vi "saveSettings.vi"(8 "error in (no error)":errorcluster, 11 "TaskRef in":refnum<vi>) -> (0 "error out":errorcluster, 3 "TaskRef out":refnum<vi>)   [LabVIEW 2015, in "pdbm_tasks.lvlib"]
doc: "saves current value of controls on VI to file. The setting file is placed in Config folder in application root folder and named as below rule thumb: <b><VI_Name>_setting.xml</b>"
uses:
  pdbm_tasks.lvlib
  <vilib>/Utility/error.llb/DialogType.ctl
  <vilib>/NI/GXML/Utility VIs/Concatenate GXML Strings.vi
  <vilib>/NI/GXML/Generator.vi
  <vilib>/NI/GXML/Write XML to File.vi
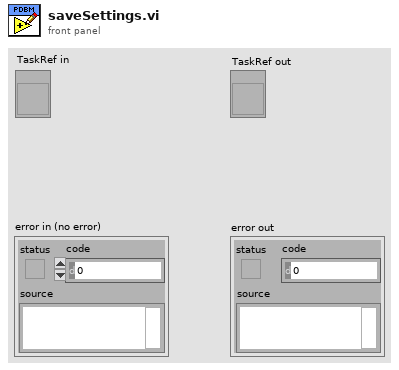
[diagram p1: front panel]
types:
  T1 = typedef "DialogType.ctl" = u16
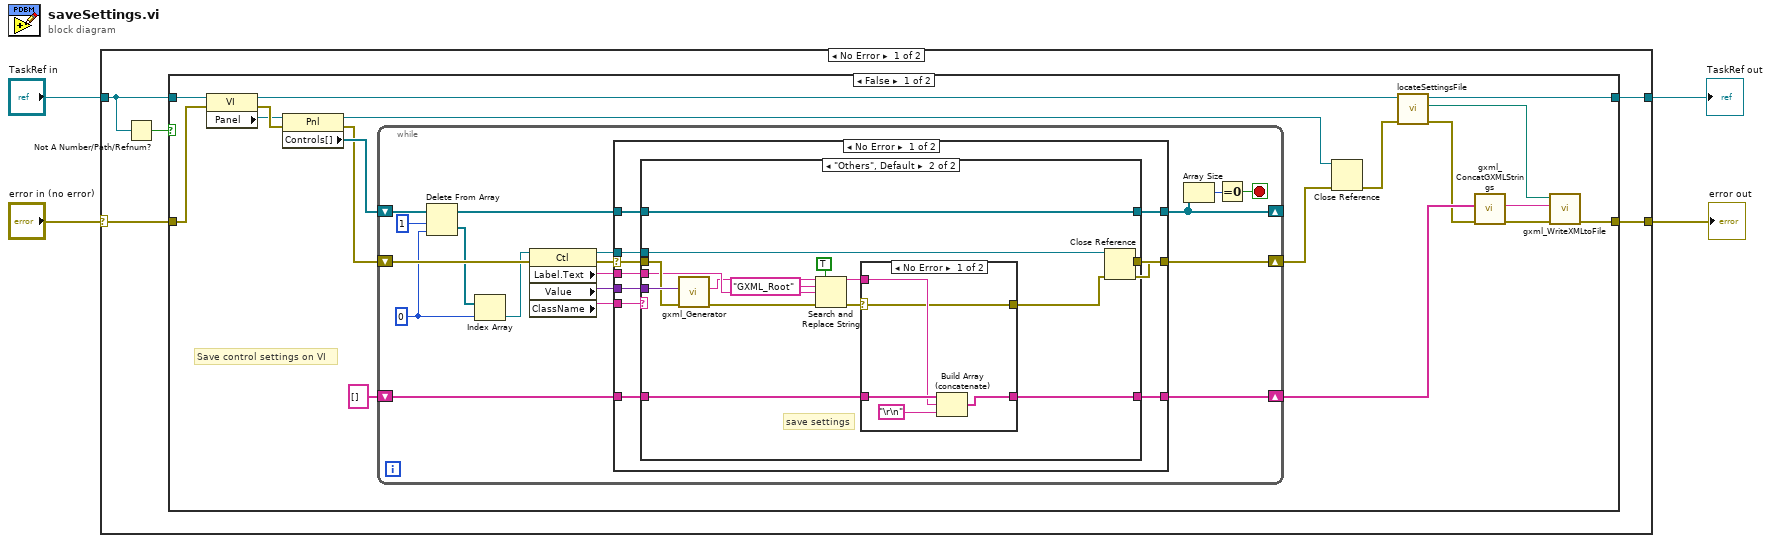
[diagram p0: block diagram]
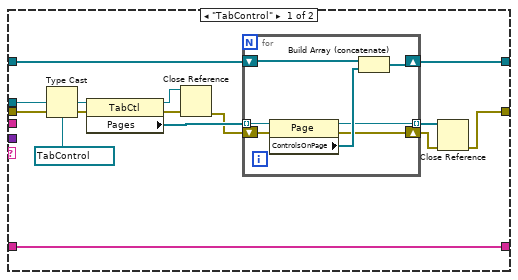
[diagram p2: hidden frame]
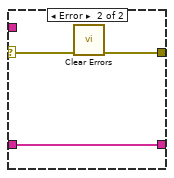
[diagram p3: hidden frame]
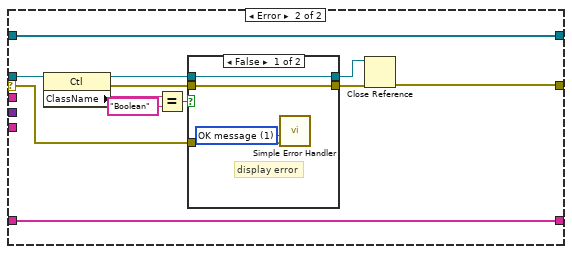
[diagram p4: hidden frame]
diagram:
  n1 = case shown="No Error" "error in (no error)" {
    selector: "error in (no error)" -> [w9 w120]
    tunnel: "TaskRef in" -> [w6 w121]
    tunnel: [w7 w121] -> w2
    tunnel: [w8 w120] -> w3
    frame No Error {
      n2 = Not A Number/Path/Refnum?(number/path/refnum=w6) -> (NaN/Path/Refnum?=w5:bool)
      n3 = case shown="False" w5 {
        tunnel: w9 -> [w27 w118]
        tunnel: [w20 w118] -> w8
        tunnel: [w15 w119] -> w7
        tunnel: w6 -> [w11 w119]
        frame False {
          # "Save control settings on VI"
          n4 = property class="VI"(reference=w11, error in=w27) -> (reference out=w16:refnum<vi>, error out=w26:errorcluster, "Panel"=w10:refnum<vi>)
          n5 = property class="Pnl"(reference=w10, error in=w26) -> (reference out=w21:refnum<vi>, error out=w24:errorcluster, "Controls[]"=w25:refnum<vi>[])
          n6 = while {
            shift-right: [w42] -> w17
            shift-left: w24 -> [w45]
            shift-right: [w38] -> w18
            shift-left: string[] [] -> [w39]
            shift-right: [w30] -> _
            shift-left: w25 -> [w36]
            stop <- w28 stop-if-true
            w31 = 0 ("index")
            n7 = Delete From Array(array=w36, length=1, index=w31) -> (deleted portion=w33:refnum<vi>[], array with subset deleted=w35:refnum<vi>[])
            n8 = Index Array(array=w33, index=w31) -> (element=w32:refnum<vi>)
            n9 = property class="Ctl"(reference=w32, error in=w45) -> (reference out=w43:refnum<vi>, error out=w44:errorcluster, "Label.Text"=w41:string, "Value"=w40:variant, "ClassName"=w37:string)
            n10 = case shown="No Error" w44 {
              selector: w44 -> [w54 w105]
              tunnel: w43 -> [w49 w109]
              tunnel: [w50 w100] -> w42
              tunnel: w41 -> [w53 _]
              tunnel: w40 -> [w55 _]
              tunnel: w39 -> [w52 w104]
              tunnel: [w51 w104] -> w38
              tunnel: w37 -> [w46 _]
              tunnel: w35 -> [w48 w103]
              tunnel: [w47 w103] -> w30
              frame No Error {
                n11 = case shown="\"Others\", Default" w46 {
                  tunnel: w55 -> [_ w91]
                  tunnel: w54 -> [w66 w90]
                  tunnel: w53 -> [_ w88]
                  tunnel: w52 -> [w69 w85]
                  tunnel: [w69 w84] -> w51
                  tunnel: [w61 w77] -> w50
                  tunnel: w49 -> [w68 w79]
                  tunnel: w48 -> [w64 w80]
                  tunnel: [w60 w80] -> w47
                  frame "TabControl" {
                    n12 = Type Cast(type=refnum<vi> refnum ("Tab Control 2"), x=w68) -> (*(type *) &x=w67:refnum<vi>)
                    n13 = property class="TabCtl"(reference=w67, error in=w66) -> (reference out=w58:refnum<vi>, error out=w59:errorcluster, "Pages"=w65:refnum<vi>[])
                    n14 = Close Reference(reference=w58, error in (no error)=w59) -> (error out=w57:errorcluster)
                    n15 = for {
                      tunnel: w65 -> [w76] mode=indexing
                      shift-right: [w72] -> w60
                      shift-left: w64 -> [w75]
                      tunnel: [w73] -> w63 mode=indexing
                      shift-right: [w71] -> w62
                      shift-left: w57 -> [w70]
                      n16 = property class="Page"(reference=w76, error in=w70) -> (reference out=w73:refnum<vi>, error out=w71:errorcluster, "ControlsOnPage"=w74:refnum<vi>[])
                      n17 = Build Array (concatenate)(w75, w74) -> (w72:refnum<vi>[])
                    }
                    n18 = Close Reference(reference=w63, error in (no error)=w62) -> (error out=w61:errorcluster)
                  }
                  frame "Others", Default {
                    # "save settings"
                    n19 = call <vilib>:"gxml_Generator.vi"("error in"=w90, "Variant"=w91) -> ("error out"=w89:errorcluster, "XML String Out"=w87:string)  [unwired: 8 in]
                    n20 = Search and Replace String(replace all?=TRUE ("replace all? (F)"), input string=w87, search string="GXML_Root", replace string=w88, error in=w89) -> (result string=w81:string, error out=w82:errorcluster)  [unwired: 3 in, 2 out]
                    n21 = case shown="No Error" w82 {
                      selector: w82 -> [w92 w99]
                      tunnel: w85 -> [w96 w97]
                      tunnel: [w95 w97] -> w84
                      tunnel: w81 -> [w93 _]
                      tunnel: [w92 w98] -> w78
                      frame No Error {
                        n22 = Build Array (concatenate)(w96, w93, "\r\n") -> (w95:string[])
                      }
                      frame Error {
                        n23 = call <vilib>:"Clear Errors.vi"("error in (no error)"=w99) -> ("error out"=w98:errorcluster)  [unwired: 5 in, 1 out]
                      }
                    }
                    n24 = Close Reference(reference=w79, error in (no error)=w78) -> (error out=w77:errorcluster)
                  }
                }
              }
              frame Error {
                n25 = property class="Ctl"(reference=w109) -> (reference out=w107:refnum<vi>, error out=w106:errorcluster, "ClassName"=w111:string)  [unwired: 1 in]
                n26 = Equal?(x=w111, y="Boolean") -> (x = y?=w108:bool)
                n27 = case shown="False" w108 {
                  tunnel: w107 -> [w115 w117]
                  tunnel: w106 -> [w112 w116]
                  tunnel: w105 -> [w114 _]
                  tunnel: [w115 w117] -> w101
                  tunnel: [w112 w116] -> w102
                  frame False {
                    w113 = T1 1 items=["no dialog", "OK message", "continue or stop message", "OK message + warnings", "continue/stop + warnings"] ("type of dialog (OK msg:1)")
                    # "display error"
                    n28 = call <vilib>:"Simple Error Handler.vi"("type of dialog (OK msg:1)"=w113, "error in (no error)"=w114) -> ()  [unwired: 3 in, 5 out]
                  }
                  frame True {
                    # "LV does not allow\nread/write this latching\nstate on Boolean control"
                  }
                }
                n29 = Close Reference(reference=w101, error in (no error)=w102) -> (error out=w100:errorcluster)
              }
            }
            n30 = Array Size(array=w30) -> (size(s)=w29:i32)
            n31 = Equal To 0?(x=w29) -> (x = 0?=w28:bool)
          }
          n32 = Close Reference(reference=w21, error in (no error)=w17) -> (error out=w13:errorcluster)
          n33 = call "locateSettingsFile.vi"("error in (no error)"=w13, "VI Refnum in"=w16) -> ("error out"=w12:errorcluster, "path"=w14:path, "VI Refnum out"=w15:refnum<vi>)  [unwired: 7 in]
          n34 = call <vilib>:"gxml_ConcatGXMLStrings.vi"("error in"=w12, "GXML Strings"=w18) -> ("error out"=w23:errorcluster, "Concatenated GXML String"=w22:string)  [unwired: 8 in]
          n35 = call <vilib>:"gxml_WriteXMLtoFile.vi"("error in"=w23, "XML Input"=w22, "XML File Path"=w14) -> ("error out"=w20:errorcluster)  [unwired: 7 in, 1 out]
        }
        frame True {
        }
      }
    }
    frame Error {
    }
  }
  "error out" <- w3
  "TaskRef out" <- w2
